vi "ValidateBarcode.vi"   [LabVIEW 2026]
uses:
  Libraries/prod_a/vision_core.dll
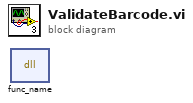
[diagram p0: block diagram]
diagram:
  n1 = dll-call lib="D:/git_proj/LabC-Vision/vision_hmi_lv/SubVIs/Libraries/prod_a/vision_core.dll" fn="func_name"() -> ()  [unwired: 6 in, 2 out]
